vi "Send Save or Load Config.vi"(1 "GUI Helper Q":refnum<queue>, 2 "Config Select Ref":refnum<vi>, 4 "Task Info in":refnum<vi>, 5 "Save?":bool, 6 "Auto Clust":refnum<vi>, 7 "Priority":T1=enum."Normal" caption="Message Priority (Normal)", 8 "error in (no error)":errorcluster, 9 "Task Configuration Name":string, 10 "Task Selection in":refnum<vi>, 11 "Message Enqueuer in":refnum<class "Message Enqueuer.lvclass">) -> (0 "error out":errorcluster, 3 "Message Enqueuer out":refnum<class "Message Enqueuer.lvclass">)   [LabVIEW 2020, in "GUI.lvlib" / "Save or Load Config Msg.lvclass"]
doc: "Sends the <b>GUI.lvlib:Save or Load Config Msg.lvclass</b> message.\n\nThis message will call <b>Save or Load Config.vi</b> on the <b>GUI.lvlib:GUI.lvclass</b> actor.\n\n<b>Save or Load Config.vi Description</b>"
uses:
  Save or Load Config Msg.lvclass
  <vilib>/ActorFramework/Message Enqueuer/Message Enqueuer.lvclass
  <vilib>/ActorFramework/Message Enqueuer/Message Priority.ctl
  Task selection df.ctl
  Automate df.ctl
  Task info df.ctl
  GUI/Task Active Enum df.ctl
  C:/Program Files/National Instruments/LabVIEW 2020/vi.lib/ActorFramework/Message/Message.lvclass
  Save or Load Config Msg.lvclass/Save or Load Config Msg.ctl
  <vilib>/ActorFramework/Message Enqueuer/Message Enqueuer.lvclass/Message Enqueuer.ctl
  <vilib>/ActorFramework/Message Priority Queue/Priority Enqueue.vi
panel:
  # "Left Arm"
  # "Right Arm"
  # "Patterns"
  # "Phase"
  # "Left        Right"
  # "Left        Right"
  # "Input Type"
  # "Task Type"
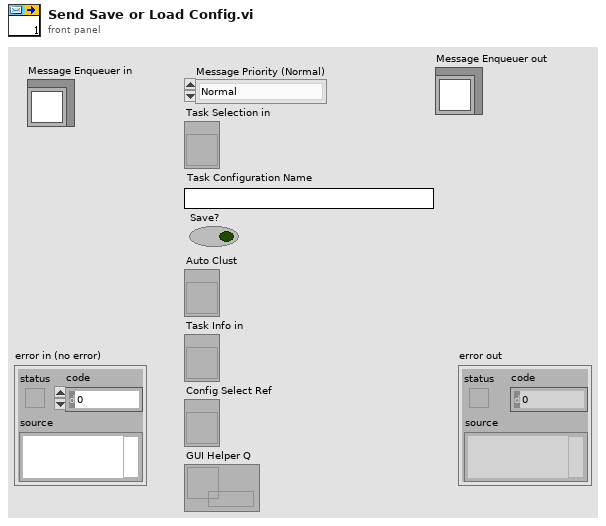
[diagram p1: front panel]
types:
  T1 = typedef "Actor Framework.lvlib/Message Enqueuer.lvclass/Message Priority.ctl" = enum16{"Low", "Normal", "High"}
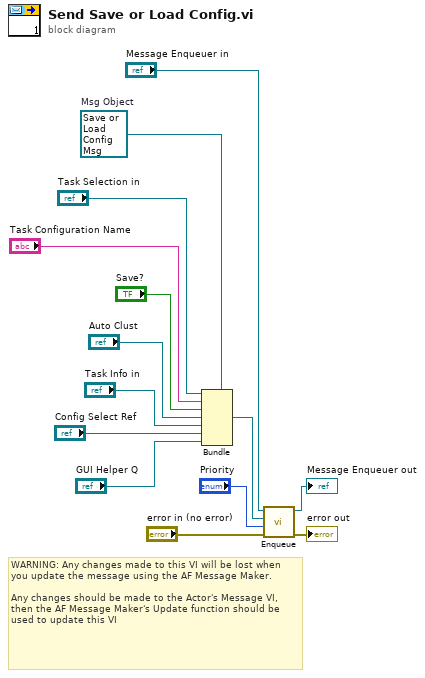
[diagram p0: block diagram]
diagram:
  w7 = refnum<class "Save or Load Config Msg.lvclass"> refnum  # Msg Object
  # "WARNING: Any changes made to this VI will be lost when you update the message using the AF Message Maker.\n\nAny changes should be made to the Actor's Message VI, then the AF Message Maker's Update function should be used to update this VI"
  n1 = Bundle(cluster=w7, "Task Selection in", "Task Configuration Name", "Save?", "Auto Clust", "Task Info in", "Config Select Ref", "GUI Helper Q") -> (w2:refnum<class "Save or Load Config Msg.lvclass">)
  n2 = call <vilib>:"Enqueue.vi"("error in (no error)"="error in (no error)", "Message Priority (Normal)"="Priority", "Message"=w2, "Message Enqueuer in"="Message Enqueuer in") -> ("error out"=→"error out":errorcluster, "Message Enqueuer out"=→"Message Enqueuer out":refnum<class "Message Enqueuer.lvclass">)  [unwired: 6 in]
